vi "rad_Configure Target.vi"(8 "error in (no error)":errorcluster, 9 "Target settings in":T1={"Hostname"="", "Serial number"="", "Product name"="", "Product code"=0, "System status"="", "Credential type"=enum."None/Unlocked", "User added?"=FALSE, "Primary NIC"={"MAC address"="", "IP Address Request Mode"=2, "IP address"="", "Subnet mask"="", "Gateway"="", "DNS server"=""}} {"Primary NIC"."IP Address Request Mode" items=["Static"=1, "DHCP/Link-Local"=2, "Link-Local Only"=4, "DHCP Only"=8]}, 11 "Target Config Options in":T3={"NumInBatch"=0, "Target Config Operation"=enum."No Config", "Target Name"="", "Increment Static IPs"=FALSE, "Change Target Name"=FALSE, "Primary NIC"={"MAC address"="", "IP Address Request Mode"=2, "IP address"="", "Subnet mask"="", "Gateway"="", "DNS server"=""}} {"Primary NIC"."IP Address Request Mode" items=["Static"=1, "DHCP/Link-Local"=2, "Link-Local Only"=4, "DHCP Only"=8]}) -> (0 "error out":errorcluster, 1 "Target settings out":T1={"Hostname"="", "Serial number"="", "Product name"="", "Product code"=0, "System status"="", "Credential type"=enum."None/Unlocked", "User added?"=FALSE, "Primary NIC"={"MAC address"="", "IP Address Request Mode"=2, "IP address"="", "Subnet mask"="", "Gateway"="", "DNS server"=""}} {"Primary NIC"."IP Address Request Mode" items=["Static"=1, "DHCP/Link-Local"=2, "Link-Local Only"=4, "DHCP Only"=8]}, 3 "Target Config Options out":T3={"NumInBatch"=0, "Target Config Operation"=enum."No Config", "Target Name"="", "Increment Static IPs"=FALSE, "Change Target Name"=FALSE, "Primary NIC"={"MAC address"="", "IP Address Request Mode"=2, "IP address"="", "Subnet mask"="", "Gateway"="", "DNS server"=""}} {"Primary NIC"."IP Address Request Mode" items=["Static"=1, "DHCP/Link-Local"=2, "Link-Local Only"=4, "DHCP Only"=8]})   [LabVIEW 2013]
uses:
  App Images/TypeDefs/rad_Target Configuration Settings.ctl
  App Images/TypeDefs/rad_Target Configuration Operations.ctl
  TypeDefs/rad_Target Network Settings.ctl
  TypeDefs/rad_Target Information.ctl
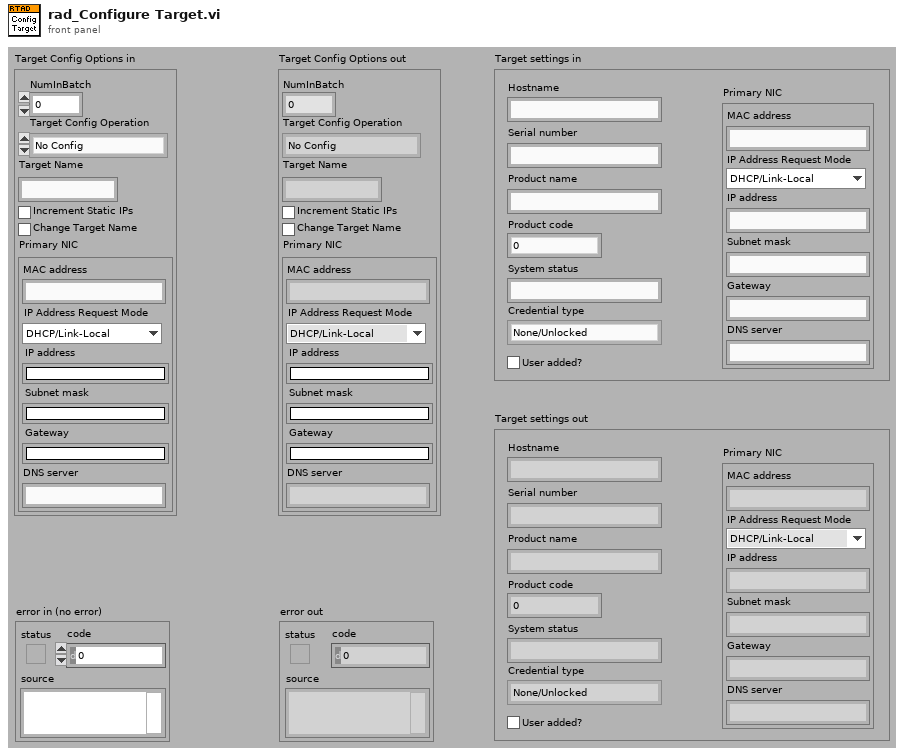
[diagram p1: front panel]
types:
  T1 = typedef "rad_Target Information.ctl" = cluster{"Hostname":string, "Serial number":string, "Product name":string, "Product code":i32, "System status":string, "Credential type":enum16{"None/Unlocked", "FTP Password", "NIAuth Credentials"}, "User added?":bool, "Primary NIC":T2}
  T2 = typedef "rad_Target Network Settings.ctl" = cluster{"MAC address":string, "IP Address Request Mode":i32, "IP address":string, "Subnet mask":string, "Gateway":string, "DNS server":string}
  T3 = typedef "rad_Target Configuration Settings.ctl" = cluster{"NumInBatch":u32, "Target Config Operation":T4, "Target Name":string, "Increment Static IPs":bool, "Change Target Name":bool, "Primary NIC":T2}
  T4 = typedef "rad_Target Configuration Operations.ctl" = enum8{"No Config", "Image Config", "Static Config"}
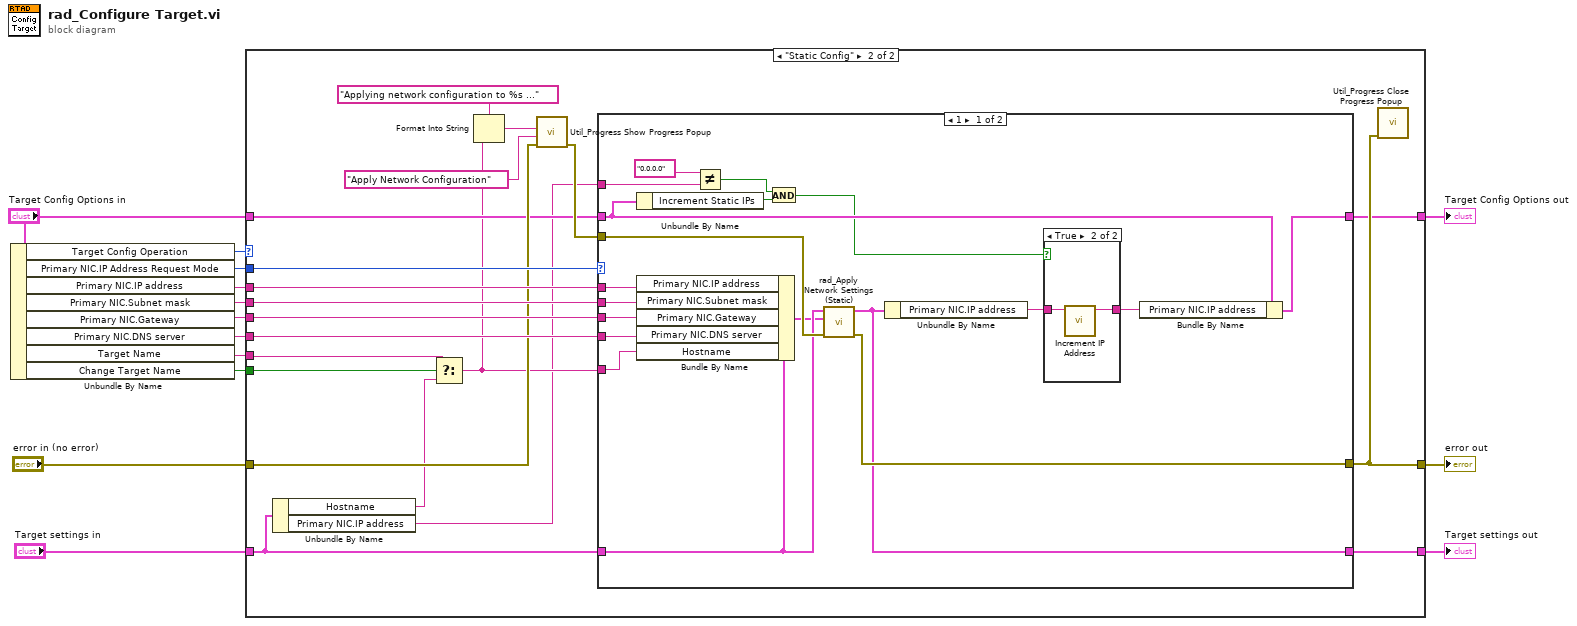
[diagram p0: block diagram]
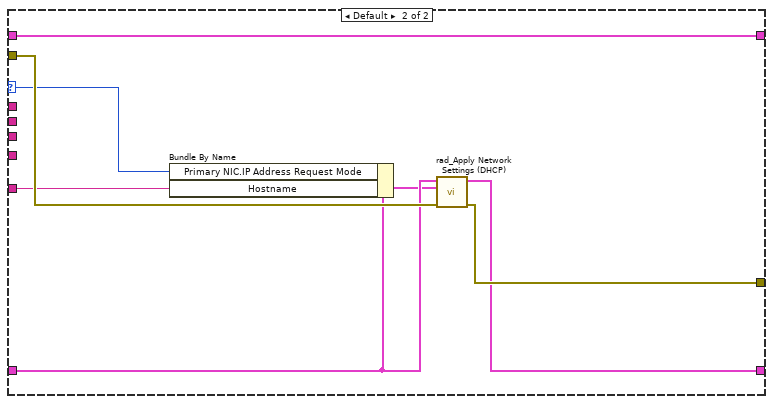
[diagram p4: hidden frame]
diagram:
  n1 = Unbundle By Name("Target Config Options in") -> ("Target Config Operation"=w14:T4, "Primary NIC.IP Address Request Mode"=w13:i32, "Primary NIC.IP address"=w12:string, "Primary NIC.Subnet mask"=w4:string, "Primary NIC.Gateway"=w11:string, "Primary NIC.DNS server"=w10:string, "Target Name"=w6:string, "Change Target Name"=w7:bool)
  n2 = case shown="\"Static Config\"" w14 {
    tunnel: w13 -> [_ w37]
    tunnel: w12 -> [_ w36]
    tunnel: w4 -> [_ w35]
    tunnel: w11 -> [_ w34]
    tunnel: w10 -> [_ w33]
    tunnel: "error in (no error)" -> [w17 w30]
    tunnel: [w17 w28] -> w8
    tunnel: w7 -> [_ w26]
    tunnel: w6 -> [_ w25]
    tunnel: "Target Config Options in" -> [w16 w24]
    tunnel: [w16 w23] -> w3
    tunnel: "Target settings in" -> [w15 w20]
    tunnel: [w15 w21] -> w1
    frame Default {
    }
    frame "Static Config" {
      n3 = Unbundle By Name(w20) -> ("Hostname"=w18:string, "Primary NIC.IP address"=w19:string)
      n4 = Select(t=w25, s=w26, f=w18) -> (s? t:f=w22:string)
      n5 = Format Into String(format string="Applying network configuration to %s ..." ("Message"), w22) -> (resulting string=w31:string)  [unwired: 2 in, 1 out]
      n6 = call "Util_Progress Show Progress Popup.vi"("error in (no error)"=w30, "Title"="Apply Network Configuration", "Message"=w31) -> ("error out"=w27:errorcluster)  [unwired: 8 in]
      n7 = case shown="1" w37 {
        selector: w37 -> [_ w60]
        tunnel: w36 -> [w56 _]
        tunnel: w35 -> [w55 _]
        tunnel: w34 -> [w54 _]
        tunnel: w33 -> [w53 _]
        tunnel: [w43 w67] -> w28
        tunnel: w27 -> [w52 w66]
        tunnel: w19 -> [w51 _]
        tunnel: w24 -> [w47 w65]
        tunnel: [w46 w65] -> w23
        tunnel: w22 -> [w44 w63]
        tunnel: w20 -> [w39 w62]
        tunnel: [w40 w64] -> w21
        frame 1 {
          n8 = Unbundle By Name(w47) -> ("Increment Static IPs"=w49:bool)
          n9 = Bundle By Name(cluster=w39, "Primary NIC.IP address"=w56, "Primary NIC.Subnet mask"=w55, "Primary NIC.Gateway"=w54, "Primary NIC.DNS server"=w53, "Hostname"=w44) -> (w38:T1)
          n10 = Not Equal?(x="0.0.0.0" ("y"), y=w51) -> (x != y?=w48:bool)
          n11 = And(x=w48, y=w49) -> (x .and. y?=w45:bool)
          n12 = call "rad_Apply Network Settings (Static).vi"("error in (no error)"=w52, "Requested settings"=w38, "Existing settings"=w39) -> ("error out"=w43:errorcluster, "Target settings out"=w40:T1)  [unwired: 7 in]
          n13 = Unbundle By Name(w40) -> ("Primary NIC.IP address"=w41:string)
          n14 = case shown="True" w45 {
            tunnel: w41 -> [w57 w59]
            tunnel: [w57 w58] -> w42
            frame False {
            }
            frame True {
              n15 = call "Increment IP Address.vi"("IP Address"=w59) -> ("New IP Address"=w58:string)  [unwired: 8 in, 2 out]
            }
          }
          n16 = Bundle By Name(cluster=w47, "Primary NIC.IP address"=w42) -> (w46:T3)
        }
        frame Default {
          n17 = Bundle By Name(cluster=w62, "Primary NIC.IP Address Request Mode"=w60, "Hostname"=w63) -> (w61:T1)
          n18 = call "rad_Apply Network Settings (DHCP).vi"("error in (no error)"=w66, "Requested settings"=w61, "Existing settings"=w62) -> ("error out"=w67:errorcluster, "Target settings out"=w64:T1)  [unwired: 7 in]
        }
      }
      n19 = call "Util_Progress Close Progress Popup.vi"("error in (no error)"=w28) -> ()  [unwired: 10 in, 1 out]
    }
  }
  "error out" <- w8
  "Target Config Options out" <- w3
  "Target settings out" <- w1
